vi "sub_qam_symbol_map_gen.vi"(9 "Gray code?":bool, 11 "M-QAM":i32) -> (3 "symbol map":cdb[](array[numeric]))   [LabVIEW 2014]
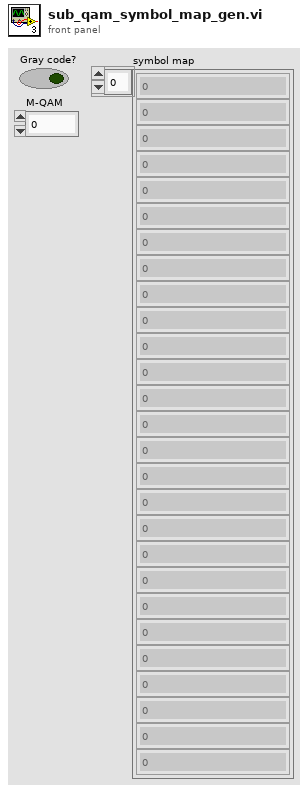
[diagram p1: front panel]
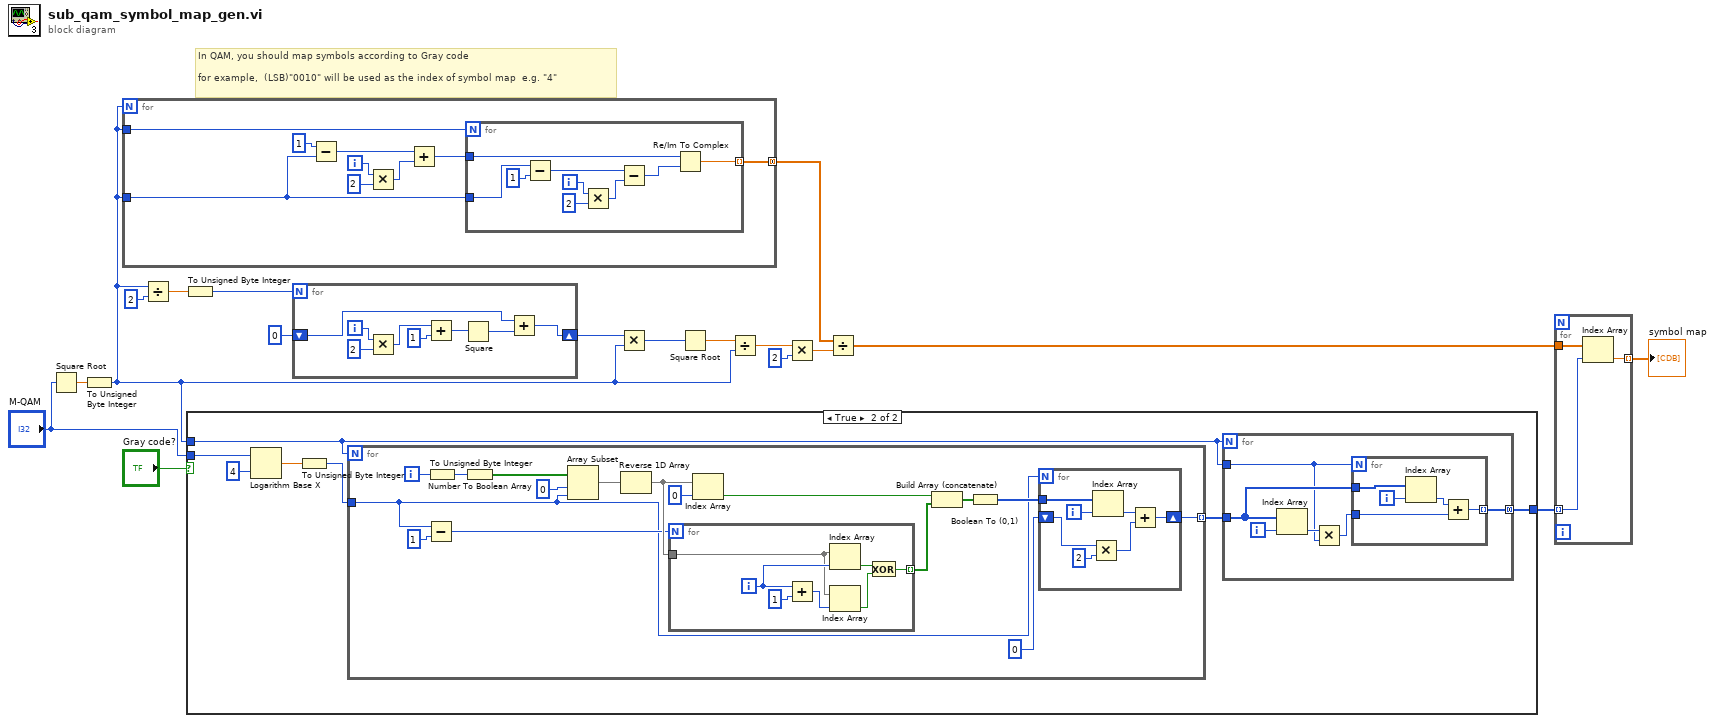
[diagram p0: block diagram]
diagram:
  # "In QAM, you should map symbols according to Gray code\n\nfor example,  (LSB)\"0010\" will be used as the index of symbol map  e.g. \"4\""
  n1 = Square Root(x="M-QAM") -> (sqrt(x)=w17:dbl)
  n2 = To Unsigned Byte Integer(number=w17) -> (unsigned 8bit integer=w4:u8)
  n3 = for {
    N: w4 -> [_]
    tunnel: w4 -> [w22]
    tunnel: [w25] -> w11 mode=concatenating
    tunnel: w4 -> [w24]
    i -> [w27]
    n4 = Subtract(x=1, y=w22) -> (x-y=w20:i32)
    n5 = Multiply(x=w27, y=2) -> (x*y=w19:i32)
    n6 = Add(x=w20, y=w19) -> (x+y=w21:i32)
    n7 = for {
      N: w24 -> [_]
      tunnel: w21 -> [w29]
      tunnel: w22 -> [w30]
      tunnel: [w34] -> w25 mode=indexing
      i -> [w36]
      n8 = Subtract(x=w30, y=1) -> (x-y=w33:i32)
      n9 = Multiply(x=w36, y=2) -> (x*y=w32:i32)
      n10 = Subtract(x=w33, y=w32) -> (x-y=w28:i32)
      n11 = Re/Im To Complex(1:w28, 2:w29) -> (0:w34:cdb)
    }
  }
  n12 = Divide(x=w4, y=2) -> (x/y=w9:dbl)
  n13 = To Unsigned Byte Integer(number=w9) -> (unsigned 8bit integer=w13:u8)
  n14 = case shown="True" "Gray code?" {
    tunnel: "M-QAM" -> [w38 w41]
    tunnel: [w37 w43] -> w16
    tunnel: w4 -> [_ w40]
    frame False {
      n15 = for {
        N: w38 -> [_]
        tunnel: [w39] -> w37 mode=indexing
        i -> [w39]
      }
    }
    frame True {
      n16 = Logarithm Base X(1:4, 2:w41) -> (0:w45:dbl)
      n17 = To Unsigned Byte Integer(number=w45) -> (unsigned 8bit integer=w42:u8)
      n18 = for {
        N: w40 -> [_]
        tunnel: w42 -> [w58]
        tunnel: [w59] -> w44 mode=indexing
        i -> [w63]
        n19 = Subtract(x=w58, y=1) -> (x-y=w68:i32)
        n20 = To Unsigned Byte Integer(number=w63) -> (unsigned 8bit integer=w64:u8)
        n21 = Number To Boolean Array(number=w64) -> (Boolean array=w66:bool[])
        n22 = Array Subset(array=w66, index=0, length=w58) -> (w71:bool[])
        n23 = Reverse 1D Array(array=w71) -> (reversed array=w72:bool[])
        n24 = for {
          N: w68 -> [_]
          tunnel: [w81] -> w70 mode=indexing
          tunnel: w72 -> [w83]
          i -> [w84]
          n25 = Add(x=w84, y=1) -> (x+y=w87:i32)
          n26 = Index Array(array=w83, index=w84) -> (element=w82:bool)
          n27 = Index Array(array=w83, index=w87) -> (element=w85:bool)
          n28 = Exclusive Or(1:w85, 2:w82) -> (0:w81:bool)
        }
        n29 = Index Array(array=w72, index=0) -> (element=w69:bool)
        n30 = Build Array (concatenate)(w69, w70) -> (w60:bool[])
        n31 = Boolean To (0,1)(Boolean=w60) -> (0, 1=w61:i16[])
        n32 = for {
          N: w58 -> [_]
          tunnel: w61 -> [w80]
          shift-right: [w75] -> w59
          shift-left: 0 -> [w76]
          i -> [w74]
          n33 = Multiply(x=w76, y=2) -> (x*y=w77:i32)
          n34 = Index Array(array=w80, index=w74) -> (element=w78:i16)
          n35 = Add(x=w78, y=w77) -> (x+y=w75:i32)
        }
      }
      n36 = for {
        N: w40 -> [_]
        tunnel: w44 -> [w50]
        tunnel: w40 -> [w47]
        tunnel: [w48] -> w43 mode=concatenating
        i -> [w52]
        n37 = Index Array(array=w50, index=w52) -> (element=w51:i32)
        n38 = Multiply(x=w51, y=w47) -> (x*y=w49:i32)
        n39 = for {
          N: w47 -> [_]
          tunnel: w50 -> [w56]
          tunnel: w49 -> [w54]
          tunnel: [w53] -> w48 mode=indexing
          i -> [w57]
          n40 = Index Array(array=w56, index=w57) -> (element=w55:i32)
          n41 = Add(x=w55, y=w54) -> (x+y=w53:i32)
        }
      }
    }
  }
  n42 = for {
    N: w13 -> [_]
    shift-right: [w90] -> w8
    shift-left: 0 -> [w88]
    i -> [w95]
    n43 = Multiply(x=w95, y=2) -> (x*y=w93:i32)
    n44 = Add(x=w93, y=1) -> (x+y=w91:i32)
    n45 = Square(x=w91) -> (x^2=w89:i32)
    n46 = Add(x=w88, y=w89) -> (x+y=w90:i32)
  }
  n47 = Multiply(x=w8, y=w4) -> (x*y=w7:i32)
  n48 = Square Root(x=w7) -> (sqrt(x)=w5:dbl)
  n49 = Divide(x=w5, y=w4) -> (x/y=w3:dbl)
  n50 = Multiply(x=w3, y=2) -> (x*y=w1:dbl)
  n51 = Divide(x=w11, y=w1) -> (x/y=w10:cdb[])
  n52 = for {
    tunnel: w16 -> [w97] mode=indexing
    tunnel: w10 -> [w98]
    tunnel: [w96] -> w15 mode=indexing
    n53 = Index Array(array=w98, index=w97) -> (element=w96:cdb)
  }
  "symbol map" <- w15
